vi "ex1_1.vi"() -> ()   [LabVIEW 2017]
panel:
  out "Temperature":dbl
  in  "Kelvin/Farneheit":bool
  in  "Celcius temperature":dbl
  # "Kelvin"
  # "Farenheit"
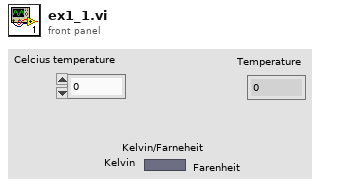
[diagram p1: front panel]
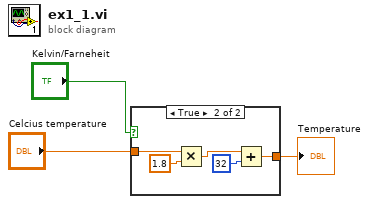
[diagram p0: block diagram]
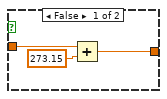
[diagram p2: hidden frame]
diagram:
  n1 = case shown="True" "Kelvin/Farneheit" {
    tunnel: "Celcius temperature" -> [w5 w9]
    tunnel: [w4 w7] -> w1
    frame False {
      n2 = Add(x=w5, y=273.15) -> (x+y=w4:dbl)
    }
    frame True {
      n3 = Multiply(x=w9, y=1.8) -> (x*y=w11:dbl)
      n4 = Add(x=w11, y=32) -> (x+y=w7:dbl)
    }
  }
  "Temperature" <- w1
